vi "Set Disk Piston.vi"(0 "Boolean":bool) -> ()   [LabVIEW 2012]
uses:
  <vilib>/Rock Robotics/WPI/Solenoid/WPI_SolenoidValue.ctl
  <vilib>/Rock Robotics/WPI/Solenoid/WPI_SolenoidSetEnum.vi
  Robot Global Data.vi
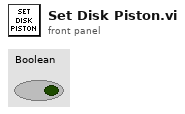
[diagram p1: front panel]
types:
  T1 = typedef "WPI_SolenoidValue.ctl" = enum16{"Off", "On", "Forward", "Reverse"}
  T2 = typedef "WPI_SolenoidDevRef.ctl" = cluster{"DevStatus":errorcluster, "Solenoid Module":T3, "Forward Solenoid Channel":T4, "Reverse Solenoid Channel":T4}
  T3 = typedef "FPGA_TypedefSolenoidModule.ctl" = enum16{"Solenoid Module 1", "Solenoid Module 2"}
  T4 = typedef "WPI_SolenoidChannel.ctl" = enum8{"Solenoid 1", "Solenoid 2", "Solenoid 3", "Solenoid 4", "Solenoid 5", "Solenoid 6", "Solenoid 7", "Solenoid 8", "Invalid"}
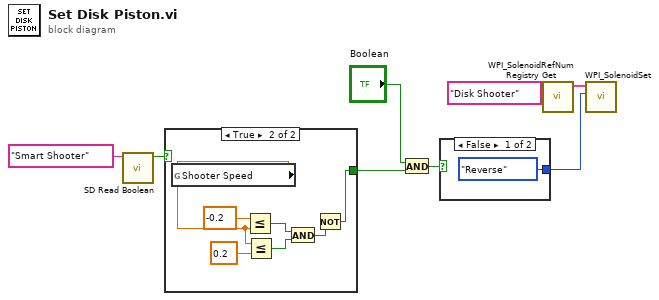
[diagram p0: block diagram]
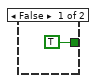
[diagram p2: hidden frame]
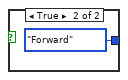
[diagram p3: hidden frame]
diagram:
  n1 = call <vilib>:"SD Read Boolean.vi"("Name"="Smart Shooter") -> ("Boolean"=w4:bool)  [unwired: 8 in, 2 out]
  n2 = case shown="True" w4 {
    tunnel: [TRUE w10] -> w1
    frame False {
    }
    frame True {
      n3 = global read "Robot Global Data.vi" "Shooter Speed"() -> (w16:dbl)
      n4 = Less Or Equal?(x=-0.2, y=w16) -> (x <= y?=w13:bool)
      n5 = Less Or Equal?(x=w16, y=0.2) -> (x <= y?=w12:bool)
      n6 = And(x=w13, y=w12) -> (x .and. y?=w11:bool)
      n7 = Not(x=w11) -> (.not. x?=w10:bool)
    }
  }
  n8 = And(x="Boolean", y=w1) -> (x .and. y?=w2:bool)
  n9 = case shown="False" w2 {
    tunnel: [WPI_SolenoidValue."Reverse" ("Value") WPI_SolenoidValue."Forward" ("Value")] -> w6
    frame False {
    }
    frame True {
    }
  }
  n10 = call <vilib>:"WPI_SolenoidRefNum Registry Get.vi"("refnum name"="Disk Shooter") -> ("SolenoidDevRef"=w7:T2)  [unwired: 9 in, 1 out]
  n11 = call-poly <vilib>:"WPI_SolenoidSet.vi"("Value"=w6, "SolenoidDevRef"=w7) -> ()  [unwired: 8 in, 2 out]
